vi "getFlags.vi"(11 "ControlPacket in":refnum<class "ControlPacket.lvclass">) -> (0 "RETAIN":bool, 1 "QoS":T1, 2 "DUP":bool, 3 "ControlPacket out":refnum<class "ControlPacket.lvclass">)   [LabVIEW 2013, in "MQTT_Control_Packets.lvlib" / "ControlPacket.lvclass"]
uses:
  ControlPacket.lvclass
  QualityOfService -- enum.ctl
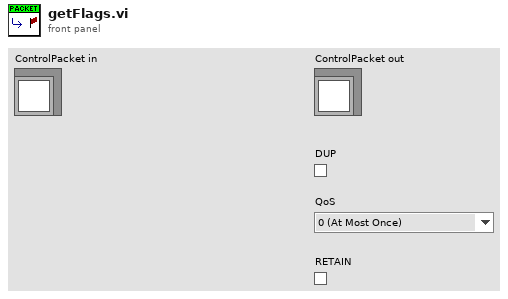
[diagram p1: front panel]
types:
  T1 = typedef "MQTT_Control_Packets.lvlib/ControlPacket.lvclass/QualityOfService -- enum.ctl" = enum16{"0 (At Most Once)", "1 (At Least Once)", "2 (Exactly Once)"}
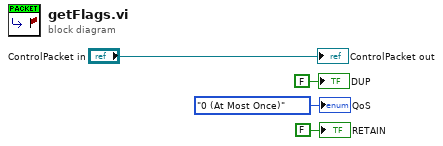
[diagram p0: block diagram]
diagram:
  "ControlPacket out" <- "ControlPacket in"
  "QoS" <- QualityOfService_--_enum."0 (At Most Once)" ("QoS")
  "DUP" <- FALSE ("DUP")
  "RETAIN" <- FALSE ("RETAIN")
